vi "closeSession.vi"(8 "error in":errorcluster, 11 "Python en entrée":refnum<class "Python.lvclass">) -> (0 "error out":errorcluster caption="sortie d'erreur", 3 "Python en sortie":refnum<class "Python.lvclass">)   [LabVIEW 2020, in "Python.lvclass"]
doc: "Close the python session.\nThis VI is mandatory."
uses:
  Python.lvclass
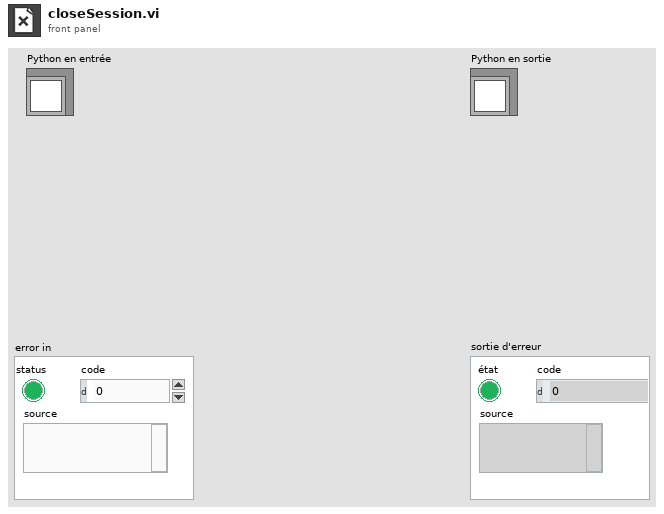
[diagram p1: front panel]
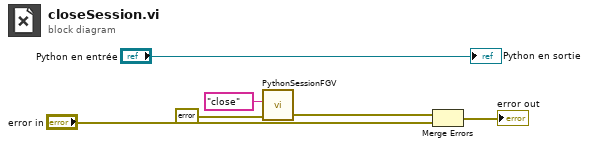
[diagram p0: block diagram]
diagram:
  n1 = call "PythonSessionFGV.vi"("error in"=errorcluster {"status"=FALSE, "code"=0, "source"=""}, "state"="close") -> ("error out"=w3:errorcluster)  [unwired: 8 in, 1 out]
  n2 = Merge Errors(w3, "error in") -> (→"error out":errorcluster)
  "Python en sortie" <- "Python en entrée"
